vi "Loop_ACT_Left_Sole.vi"() -> ()   [LabVIEW 2017, in "Claw.lvlib"]
uses:
  Claw.lvlib
  <vilib>/Rock Robotics/WPI/Solenoid/WPI_SolenoidValue.ctl
  Globals/Global_Device_IDs.vi
  <vilib>/Rock Robotics/WPI/Solenoid/WPI_SolenoidOpenSingle.vi
  _SHARE ALL/Global Share All/Global_STOP.vi
  Global_SM Write_Data Out.vi
  <vilib>/Rock Robotics/WPI/Solenoid/WPI_SolenoidSetEnum.vi
  <vilib>/Rock Robotics/WPI/Solenoid/WPI_SolenoidGetEnum.vi
  Global_ACT Write_Data Out.vi
panel:
  out "Piston Output":T1
  out "Piston Input":T1
  out "Cycle Time (S)":dbl format="%.3g"
  in  "Target Time(ms)":u32=50
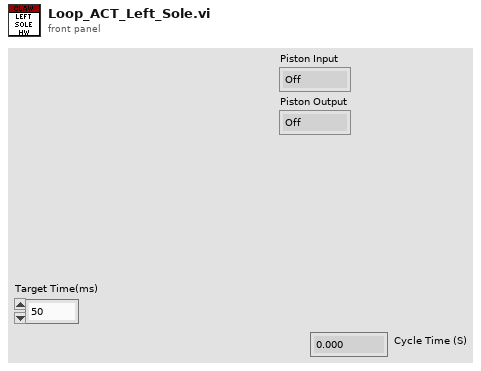
[diagram p1: front panel]
types:
  T1 = typedef "WPI_SolenoidValue.ctl" = enum16{"Off", "On", "Forward", "Reverse"}
  T2 = typedef "CLUSTER_Claw_Setup.ctl" = cluster{"Left Solenoid":T3, "Right Solenoid":T3, "Left Talon Setup":T5, "Right Talon Setup":T5}
  T3 = typedef "CLUSTER_Solonoid_Setup.ctl" = cluster{"Pneumatics Control Module (0)":u8, "Solenoid Channel":T4}
  T4 = typedef "WPI_SolenoidChannel.ctl" = enum8{"Solenoid 0", "Solenoid 1", "Solenoid 2", "Solenoid 3", "Solenoid 4", "Solenoid 5", "Solenoid 6", "Solenoid 7", "Invalid"}
  T5 = typedef "CLUSTER_Talon_Setup.ctl" = cluster{"Talon SRX ID":u8, "PhaseSensor":bool, "Invert Motor?":bool, "Phoenix Feedback Select":T6, "pidLoopldx":i32, "PID":T7}
  T6 = typedef "CTRE_Phoenix_MotorControl_FeedbackDevice.ctl" = i8
  T7 = typedef "CLUSTER_PID.ctl" = cluster{"P":dbl, "I":dbl, "D":dbl, "F":dbl, "I Zone":dbl}
  T8 = typedef "WPI_SolenoidDevRef.ctl" = cluster{"DevStatus":errorcluster, "Pneumatics Control Module":u8, "Forward Solenoid Channel":T4, "Reverse Solenoid Channel":T4}
  T9 = cluster{"SolenoidDevRef":T8, "Piston Output":T1, "Piston Input":T1, "Target Time(ms)":u32, "Current Time":timestamp, "Previous Time":timestamp, "Cycle Time (S)":dbl}
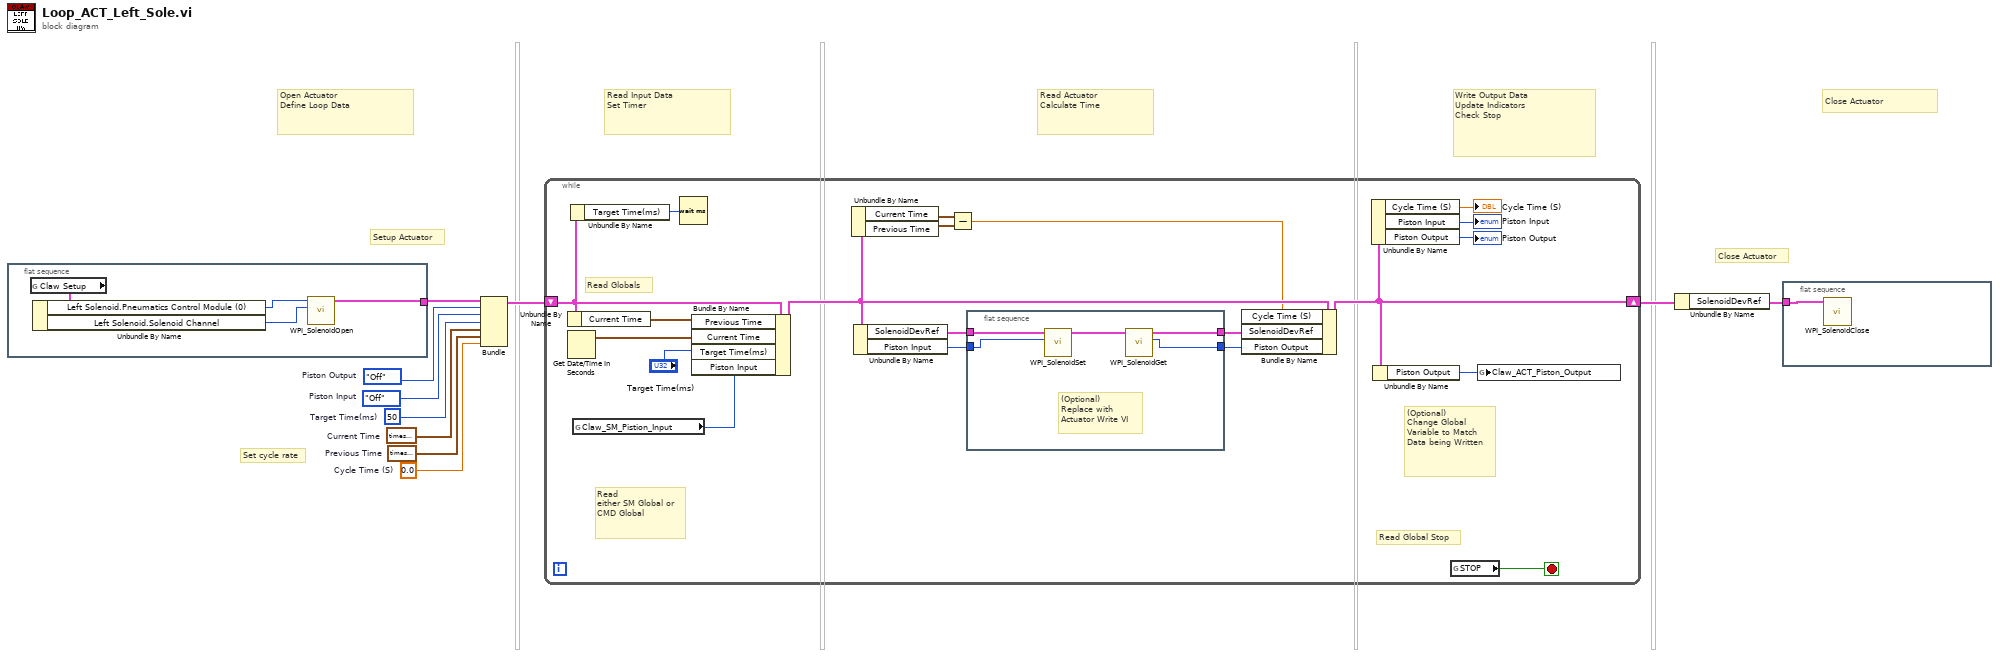
[diagram p0: block diagram]
diagram:
  w1 = WPI_SolenoidValue."Off"  # Piston Input
  w2 = WPI_SolenoidValue."Off"  # Piston Output
  w3 = 0.0  # Cycle Time (S)
  w10 = timestamp(0 s since 1904-01-01)  # Previous Time
  w9 = timestamp(0 s since 1904-01-01)  # Current Time
  w8 = u32 50  # Target Time(ms)
  # "Close Actuator"
  # "Write Output Data\nUpdate Indicators\nCheck Stop"
  # "Read Actuator\nCalculate Time"
  # "Read Input Data\nSet Timer"
  # "Open Actuator\nDefine Loop Data"
  # "Set cycle rate"
  # "Close Actuator"
  # "Setup Actuator"
  n1 = flat-sequence {
    tunnel: [w14] -> w5
    frame #0 {
      n2 = global read "Global_Device_IDs.vi" "Claw Setup"() -> (w13:T2)
      n3 = Unbundle By Name(w13) -> ("Left Solenoid.Pneumatics Control Module (0)"=w12:u8, "Left Solenoid.Solenoid Channel"=w11:T4)
      n4 = call-poly <vilib>:"WPI_SolenoidOpen.vi"("Solenoid Channel"=w11, "Pneumatics Control Module (0)"=w12) -> ("SolenoidDevRef"=w14:T8)  [unwired: 8 in, 1 out]
    }
  }
  n5 = Bundle("SolenoidDevRef"=w5, "Piston Output"=w2, "Piston Input"=w1, "Target Time(ms)"=w8, "Current Time"=w9, "Previous Time"=w10, "Cycle Time (S)"=w3) -> (w6:T9)  [unwired: 1 in]
  n6 = while {
    shift-right: [w22] -> w4
    shift-left: w6 -> [w24]
    stop <- w34 stop-if-true
    # "(Optional)\nChange Global\nVariable to Match\nData being Written"
    # "Read\neither SM Global or CMD Global"
    # "Read Globals"
    # "Read Global Stop"
    n7 = Unbundle By Name(w24) -> ("Current Time"=w29:timestamp)
    n8 = Get Date/Time In Seconds() -> (seconds since 1Jan1904=w30:timestamp)
    n9 = Unbundle By Name(w24) -> ("Target Time(ms)"=w23:u32)
    n10 = global read "Global_SM Write_Data Out.vi" "Claw_SM_Pistion_Input"() -> (w16:T1)
    n11 = Wait (ms)(milliseconds to wait=w23) -> ()  [unwired: 1 out]
    n12 = Bundle By Name(cluster=w24, "Previous Time"=w29, "Current Time"=w30, "Target Time(ms)"="Target Time(ms)", "Piston Input"=w16) -> (w25:T9)
    n13 = Unbundle By Name(w25) -> ("Current Time"=w28:timestamp, "Previous Time"=w27:timestamp)
    n14 = Unbundle By Name(w25) -> ("SolenoidDevRef"=w33:T8, "Piston Input"=w31:T1)
    n15 = Subtract(x=w28, y=w27) -> (x-y=w18:dbl)
    n16 = flat-sequence {
      tunnel: w33 -> [w39]
      tunnel: [w37] -> w32
      tunnel: w31 -> [w36]
      tunnel: [w35] -> w15
      frame #0 {
        # "(Optional)\nReplace with\nActuator Write VI"
        n17 = call-poly <vilib>:"WPI_SolenoidSet.vi"("Value"=w36, "SolenoidDevRef"=w39) -> ("SolenoidDevRef"=w38:T8)  [unwired: 8 in, 1 out]
        n18 = call-poly <vilib>:"WPI_SolenoidGet.vi"("SolenoidDevRef"=w38) -> ("Value"=w35:T1, "SolenoidDevRef"=w37:T8)  [unwired: 8 in, 1 out]
      }
    }
    n19 = Bundle By Name(cluster=w25, "Cycle Time (S)"=w18, "SolenoidDevRef"=w32, "Piston Output"=w15) -> (w22:T9)
    n20 = Unbundle By Name(w22) -> ("Cycle Time (S)"=→"Cycle Time (S)":dbl, "Piston Input"=→"Piston Input":T1, "Piston Output"=→"Piston Output":T1)
    n21 = Unbundle By Name(w22) -> ("Piston Output"=w17:T1)
    n22 = global read "Global_STOP.vi" "STOP"() -> (w34:bool)
    n23 = global write "Global_ACT Write_Data Out.vi" "Claw_ACT_Piston_Output"(w17) -> ()
  }
  n24 = Unbundle By Name(w4) -> ("SolenoidDevRef"=w7:T8)
  n25 = flat-sequence {
    tunnel: w7 -> [w40]
    frame #0 {
      n26 = call <vilib>:"WPI_SolenoidClose.vi"("SolenoidDevRef"=w40) -> ()  [unwired: 10 in, 1 out]
    }
  }
